vi "Init.vi"(10 "Player ID":i32, 11 "TeamEffort in":refnum<class "TeamEffort.lvclass">) -> (1 "X Loc":i32, 2 "Y Loc":i32, 3 "TeamEffort out":refnum<class "TeamEffort.lvclass">)   [LabVIEW 2015, in "TeamEffort.lvclass"]
uses:
  TeamEffort.lvclass
  Grid Cluster.ctl
  Player Cluster.ctl
  Team Move Input.ctl
  Type Defs/Action Enum.ctl
  Team Move Output.ctl
  Type Defs/Direction Enum.ctl
  Square/Square.lvclass
  TeamEffort.lvclass/TeamEffort.ctl
  SubVIs/Read-Only Globals.vi
  Type Defs/SB Type Defs.lvlib
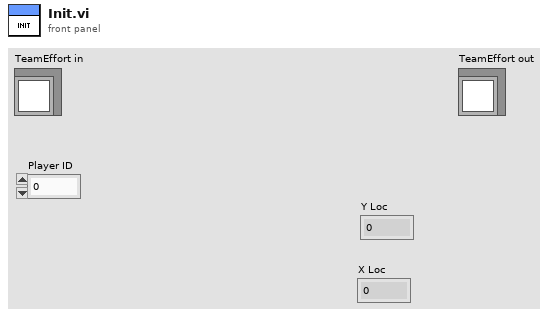
[diagram p1: front panel]
types:
  T1 = typedef "TeamEffort.lvclass/Player Cluster.ctl" = cluster{"Exp. Move":i32, "Moved?":bool, "In":T2, "Out":T4}
  T2 = typedef "TeamEffort.lvclass/Team Move Input.ctl" = cluster{"PlayerID":i32, "Y":i32, "X":i32, "Last Move":i32, "LastAction":T3}
  T3 = typedef "SB Type Defs.lvlib/Action Enum.ctl" = enum16{"Wait", "Move", "Attack", "Replicate"}
  T4 = typedef "TeamEffort.lvclass/Team Move Output.ctl" = cluster{"Action":T3, "Direction":T5, "Replicated":refnum<class "Square.lvclass">}
  T5 = typedef "SB Type Defs.lvlib/Direction Enum.ctl" = enum16{"NW", "N", "NE", "E", "SE", "S", "SW", "W"}
  T6 = typedef "TeamEffort.lvclass/Grid Cluster.ctl" = cluster{"p[x][y]":i32[][], "Move Count":i32, "Info[p]":T1[], "Known_p":i32}
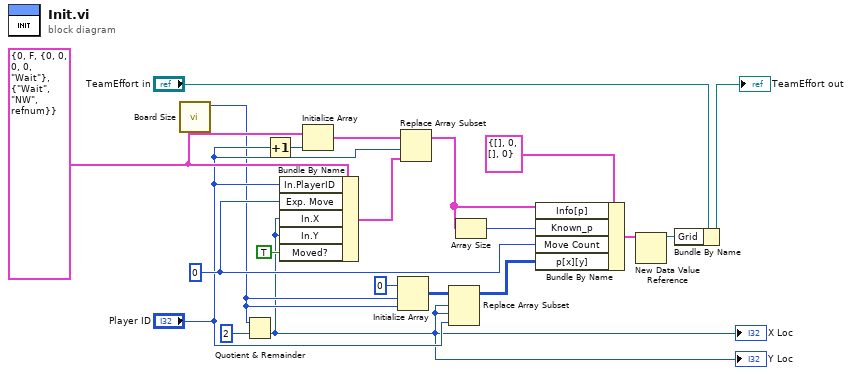
[diagram p0: block diagram]
diagram:
  w12 = T1 {"Exp. Move"=0, "Moved?"=FALSE, "In"={"PlayerID"=0, "Y"=0, "X"=0, "Last Move"=0, "LastAction"=enum."Wait"}, "Out"={"Action"=enum."Wait", "Direction"=enum."NW", "Replicated"=refnum}} ("Player Info")
  w19 = 0 ("Move Count")
  n1 = call "Board Size.vi"() -> ("Board Size"=w3:i32)  [unwired: 11 in]
  n2 = Quotient & Remainder(x=w3, y=2) -> (floor(x/y)=w1:i32)  [unwired: 1 out]
  "X Loc" <- w1
  "Y Loc" <- w1
  n3 = Increment(x="Player ID") -> (x+1=w13:i32)
  n4 = Bundle By Name(cluster=w12, "In.PlayerID"="Player ID", "Exp. Move"=w19, "In.X"=w1, "In.Y"=w1, "Moved?"=TRUE) -> (w10:T1)
  n5 = Initialize Array(w12, w13) -> (w11:T1[])
  n6 = Initialize Array(0, w3, w3) -> (w16:i32[][])
  n7 = Replace Array Subset(array=w11, new element=w10, index="Player ID") -> (w6:T1[])
  n8 = Replace Array Subset(array=w16, new element="Player ID", index (row)=w1, index (col)=w1) -> (w15:i32[][])
  n9 = Array Size(array=w6) -> (size(s)=w5:i32)
  n10 = Bundle By Name(cluster=T6 {"p[x][y]"=[], "Move Count"=0, "Info[p]"=[], "Known_p"=0} ("Grid"), "Info[p]"=w6, "Known_p"=w5, "Move Count"=w19, "p[x][y]"=w15) -> (w18:T6)
  n11 = New Data Value Reference(data value=w18) -> (data value reference=w17:refnum<data-value>)  [unwired: 1 in, 1 out]
  n12 = Bundle By Name(cluster="TeamEffort in", "Grid"=w17) -> (→"TeamEffort out":refnum<class "TeamEffort.lvclass">)
